vi "GPS -Get Coordinates from Address.vi"(11 "Inputs":T1={"City"="-1", "State"="", "Addr"="", "EID"=""}) -> (3 "Lat|Lng":string[][](array[string]))   [LabVIEW 2019]
uses:
  ctlAddrToGPSInputs.ctl
panel:
  out "error out":errorcluster
  out "EDI|Addr|Lat|Lng":string[](array[string])
  out "EID|Addr|Lat|Lng":string[][](array[string])
  in  "error in":errorcluster
  out "County/State":string
  out "Town/City":string
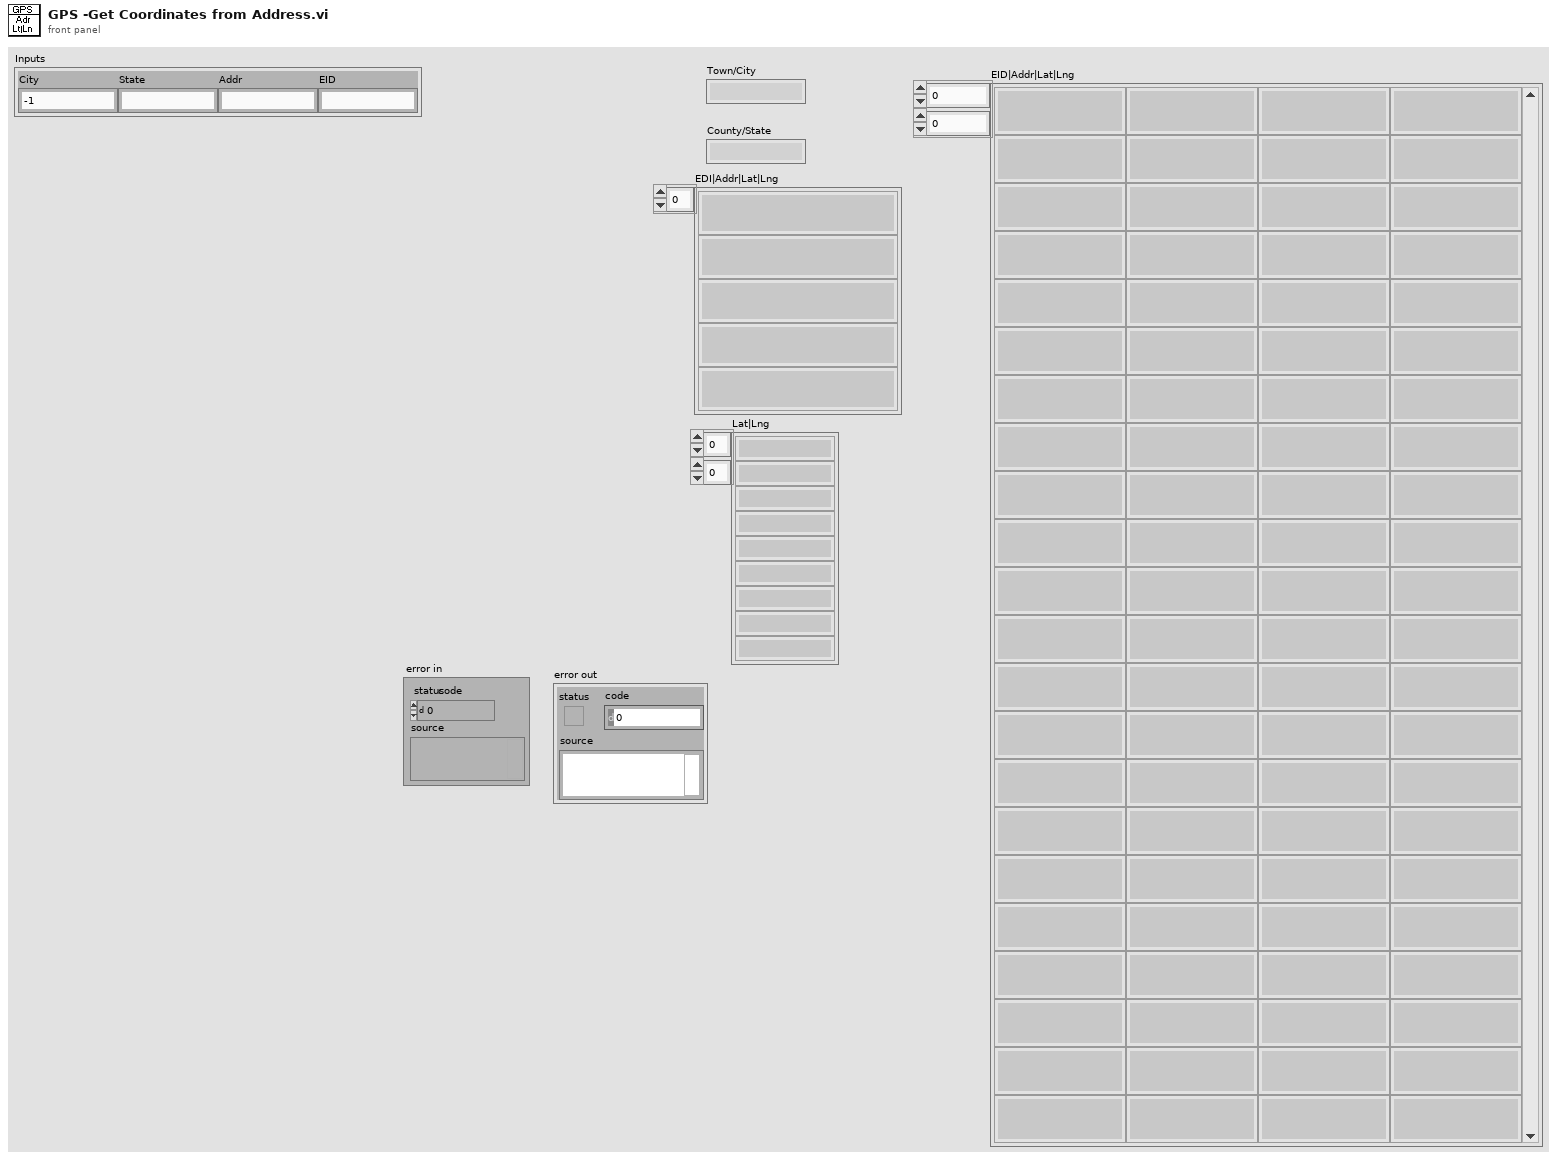
[diagram p1: front panel]
types:
  T1 = typedef "ctlAddrToGPSInputs.ctl" = cluster{"City":string, "State":string, "Addr":string, "EID":string}
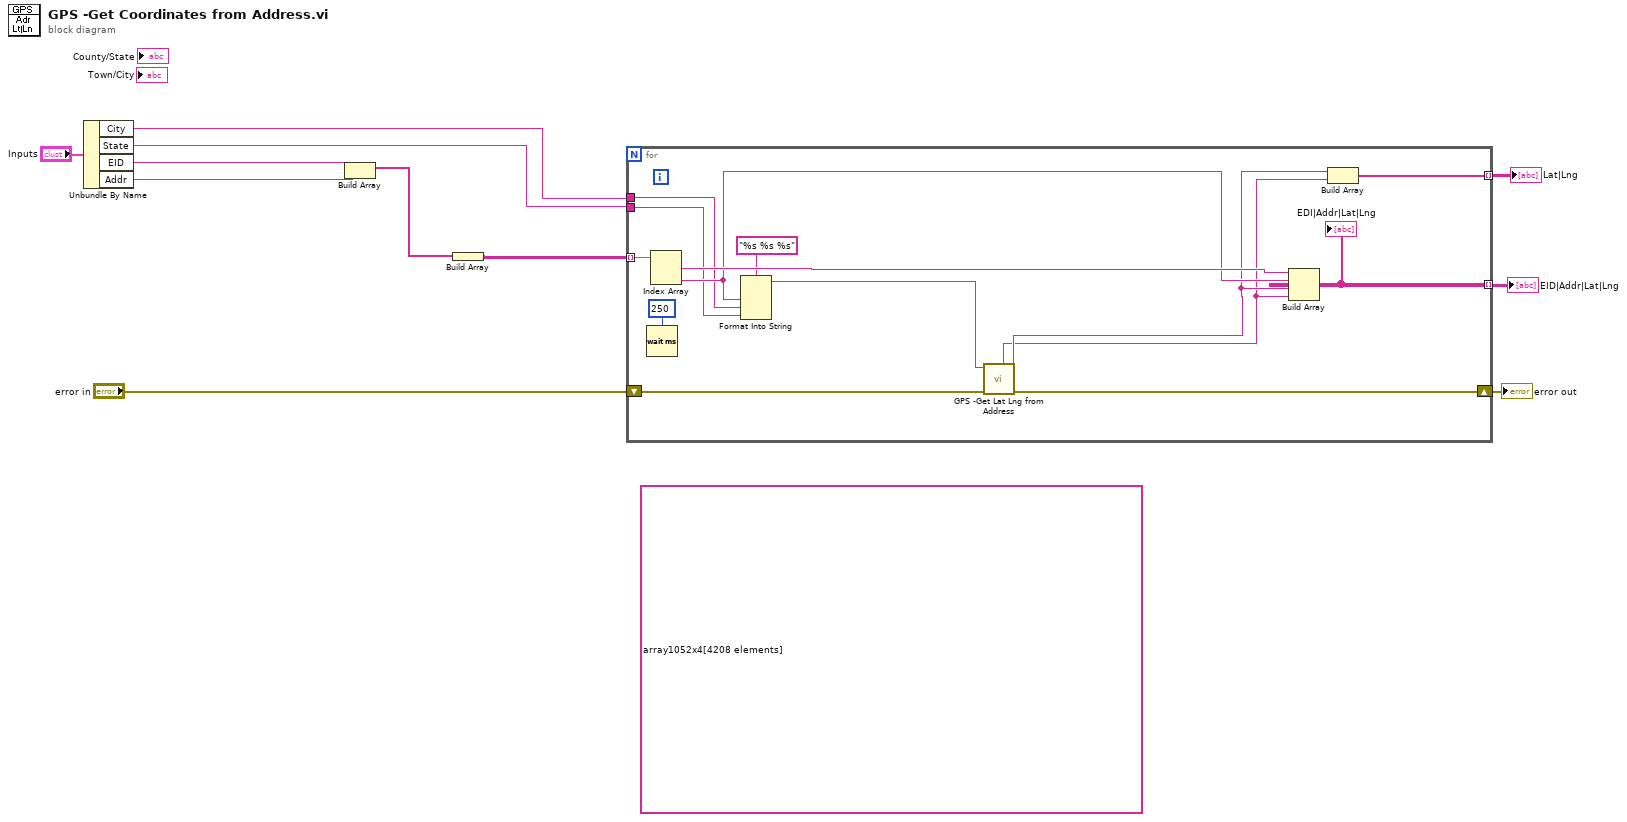
[diagram p0: block diagram]
diagram:
  (unwired) string[][] array1052x4[4208 elements] ("Array")
  n1 = Unbundle By Name("Inputs") -> ("City"=w4:string, "State"=w7:string, "EID"=w5:string, "Addr"=w6:string)
  n2 = Build Array(w5, w6) -> (w2:string[])
  n3 = Build Array(w2) -> (w10:string[][])
  n4 = for {
    shift-right: [w12] -> w1
    shift-left: "error in" -> [w13]
    tunnel: w4 -> [w18]
    tunnel: w7 -> [w17]
    tunnel: w10 -> [w25] mode=indexing
    tunnel: [w23] -> w9 mode=indexing
    tunnel: [w21] -> w3 mode=indexing
    n5 = Wait (ms)(milliseconds to wait=u32 250) -> ()  [unwired: 1 out]
    n6 = Index Array(array=w25) -> (element #1=w22:string, element #2=w19:string)  [unwired: 2 in]
    n7 = Format Into String(format string="%s %s %s", w19, w18, w17) -> (resulting string=w16:string)  [unwired: 2 in, 1 out]
    n8 = call "GPS -Get Lat Lng from Address.vi"("error in (no error)"=w13, "keywords"=w16) -> ("error out"=w12:errorcluster, "LngStrg"=w14:string, "LatStrg"=w15:string)  [unwired: 5 in, 2 out]
    n9 = Build Array(w22, w19, w15, w14) -> (w23:string[])
    "EDI|Addr|Lat|Lng" <- w23
    n10 = Build Array(w15, w14) -> (w21:string[])
  }
  "EID|Addr|Lat|Lng" <- w9
  "Lat|Lng" <- w3
  "error out" <- w1
